vi "Cluster exercise.vi"() -> ()   [LabVIEW 2018]
panel:
  in  "stop":bool
  out "Cluster 2":T1
  in  "Cluster":T1
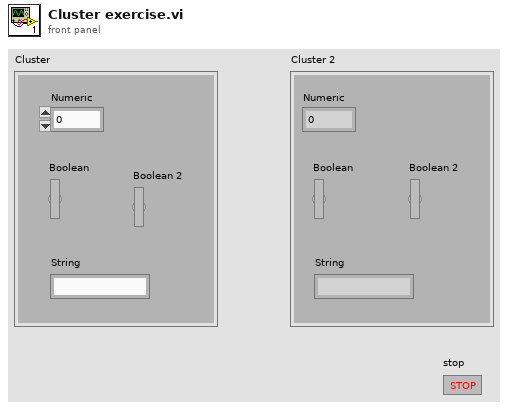
[diagram p1: front panel]
types:
  T1 = cluster{"Numeric":dbl, "Boolean":bool, "Boolean 2":bool, "String":string}
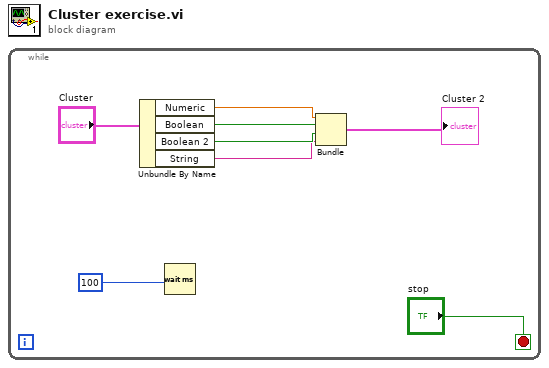
[diagram p0: block diagram]
diagram:
  n1 = while {
    stop <- "stop" stop-if-true
    n2 = Unbundle By Name("Cluster") -> ("Numeric"=w7:dbl, "Boolean"=w6:bool, "Boolean 2"=w5:bool, "String"=w4:string)
    n3 = Wait (ms)(milliseconds to wait=100) -> ()  [unwired: 1 out]
    n4 = Bundle("Numeric"=w7, "Boolean"=w6, "Boolean 2"=w5, "String"=w4) -> (→"Cluster 2":T1)  [unwired: 1 in]
  }
